vi "Project New TestCase.vi"(8 "error in (no error)":errorcluster, 11 "application reference (This Application)":refnum<vi>) -> (0 "error out":errorcluster)   [LabVIEW 2011, in "VI Tester Project API.lvlib"]
uses:
  VI Tester Project API.lvlib
  Libraries/VITesterUtilities.lvlib
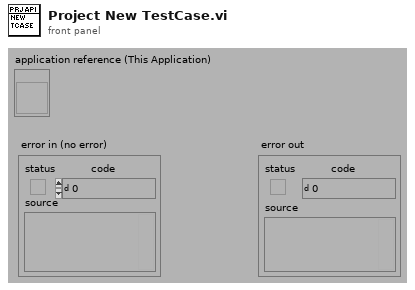
[diagram p1: front panel]
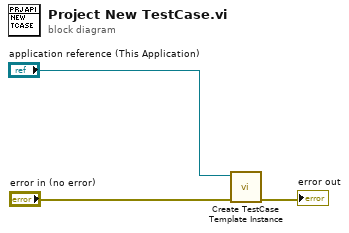
[diagram p0: block diagram]
diagram:
  n1 = call "Create TestCase Template Instance.vi"("error in"="error in (no error)", "Application Ref (This Application)"="application reference (This Application)") -> ("error out"=→"error out":errorcluster)  [unwired: 8 in, 1 out]
